vi "VisualCheck2.vi"(4 "Model":string="AVN", 6 "Slot":T1, 7 "ComPort":refnum<visa-resource-name>="COM1", 8 "error in":errorcluster, 10 "测试项":string="按键") -> (0 "error out":errorcluster, 3 "StringOut":string="ÿÿÿÿÿÿÿÿÿÿÿÿÿÿÿÿÿÿÿÿÿÿÿÿÿÿÿ")   [LabVIEW 2013]
uses:
  SystemCode/SysControl/Slot.ctl
  <vilib>/Utility/miscctls.llb/LVBoundsTypeDef.ctl
  C:/Program Files/National Instruments/LabVIEW 2013/examples/Instrument IO/Serial/support/Serial - Settings.ctl
  <vilib>/DAQmx/read.llb/DAQmx Read (Digital 1D Bool NChan 1Samp 1Line).vi
  GlobalValue.vi
  <vilib>/Instr/_visa.llb/VISA Configure Serial Port (Instr).vi
  <vilib>/DAQmx/create/channels.llb/DAQmx Create Channel (DI-Digital Input).vi
  <vilib>/DAQmx/miscellaneous.llb/DAQmx Fill In Error Info.vi
panel:
  in  "StopRef":refnum<vi>
  out "STOP2":bool
  out "按键2":T2 {"TUNE" scale=0.0..10.0}
  out "按键1":T3 {"VOL" scale=0.0..10.0}
  out "STOP":bool
  out "按键结果":bool
  out "TUNE按下":bool=TRUE
  out "TUNE旋转":bool=TRUE
  out "VOL旋转":bool=TRUE
  out "VOL按下":bool=TRUE
  out "FAIL":bool
  out "PASS":bool
  out "状态":string
  out "DVD仓":picture
  out "屏幕":picture
  in  "Debug":bool
  out "反馈结果":bool
  out "对比字符串":string
  in  "测试项目":u16(ring) items=["Reset", "按键", "倒车视频", "倒车视频", "按键灯亮", "DVD灯光红色", "DVD灯光蓝色", "按键灯亮", "入碟", "放入CD碟", "放入DVD碟", "出碟", "换碟", "视频播放", "拔除USB1", "拔除USB", "拔除导航卡", "拔除SD卡"]
  out "Result":bool
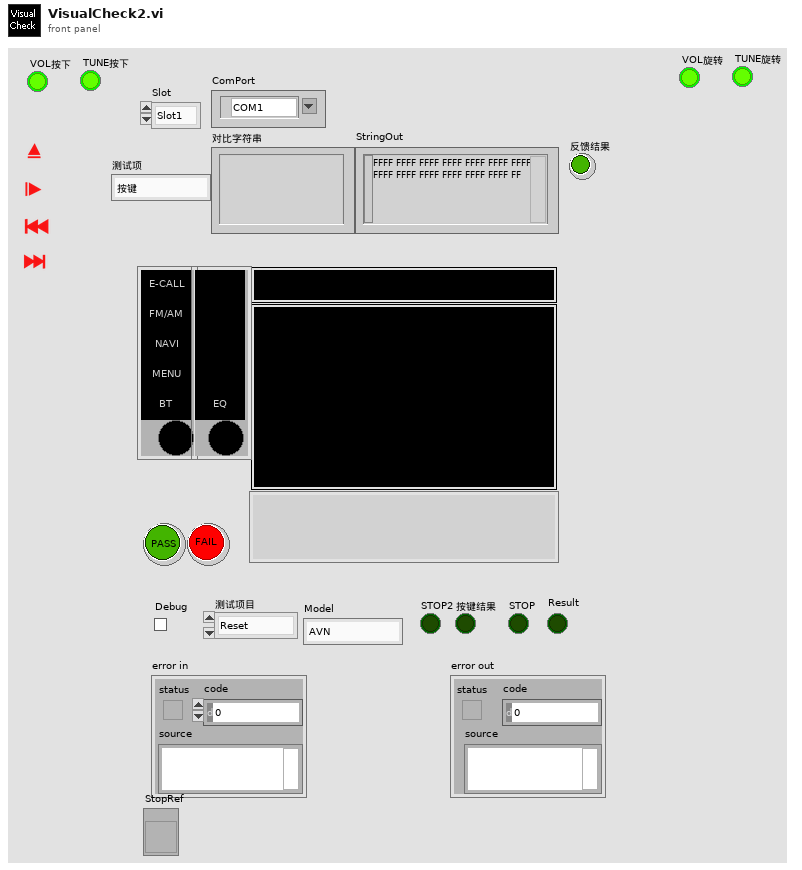
[diagram p1: front panel]
types:
  T1 = typedef "Slot.ctl" = enum16{"Slot1", "Slot2", "Slot3", "Slot4"}
  T2 = cluster{"EJECT":bool, "PLAY/PAUSE":bool, "PREV":bool, "NEXT":bool, "EQ":bool, "SRC":bool, "TUNE":dbl, "SEL":bool}
  T3 = cluster{"ECALL":bool, "FM/AM":bool, "NAVI":bool, "MENU":bool, "BT":bool, "DVD":bool, "VOL":dbl, "AUXIN":bool}
  T4 = typedef "Serial - Settings.ctl" = cluster{"波特率":u32, "数据比特":u16, "奇偶":enum16{"None", "Odd", "Even", "Mark", "Space"}, "停止位":u16, "流控制":u16}
  T5 = typedef "LVBoundsTypeDef.ctl" = cluster{"Width":u32, "Height":u32}
  T6 = typedef "DAQConfig.ctl" = cluster{"DIO":string[][], "AO":string[][], "AI":string[][]}
  T7 = typedef "imagedata.ctl" = cluster{"image type":i32, "image depth":i32, "image":u8[], "mask":u8[], "colors":u32[], "Rectangle":cluster{"left":i16, "top":i16, "right":i16, "bottom":i16}}
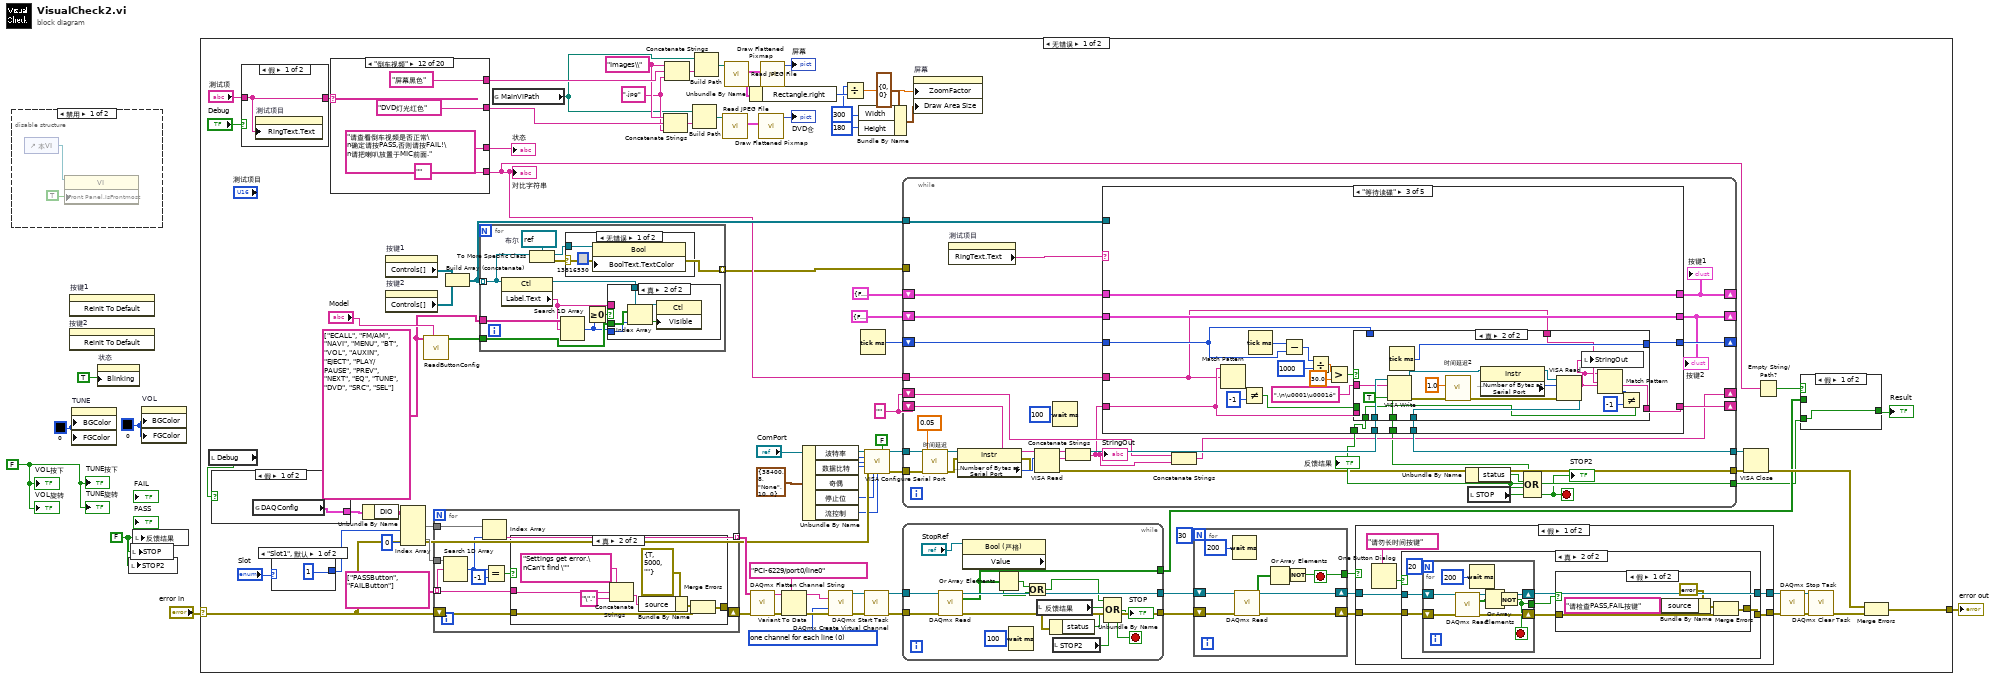
[diagram p0: block diagram]
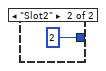
[diagram p3: hidden frame]
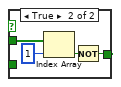
[diagram p4: hidden frame]
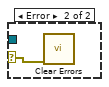
[diagram p5: hidden frame]
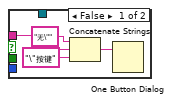
[diagram p6: hidden frame]
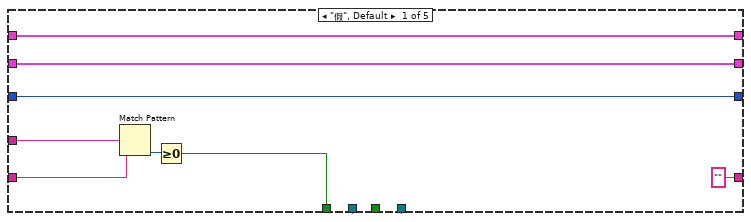
[diagram p7: hidden frame]
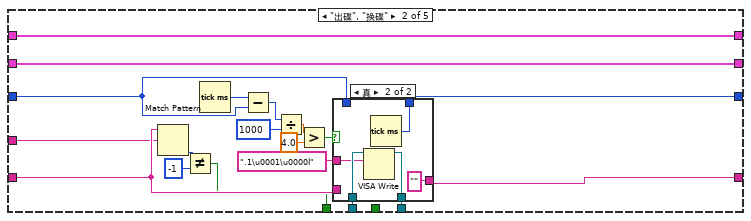
[diagram p8: hidden frame]
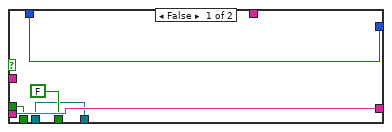
[diagram p10: hidden frame]
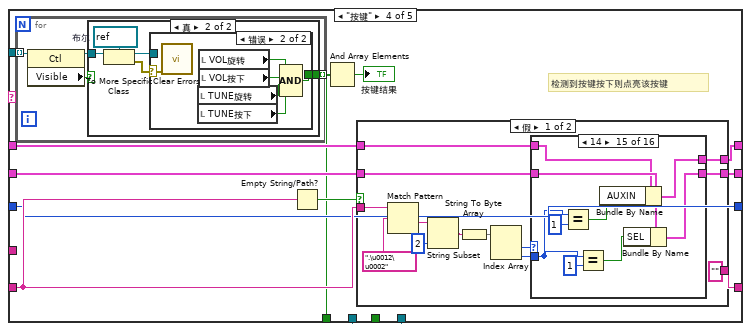
[diagram p11: hidden frame]
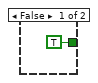
[diagram p12: hidden frame]
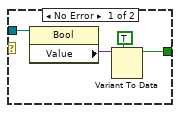
[diagram p13: hidden frame]
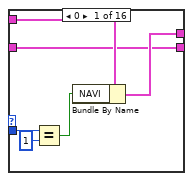
[diagram p14: hidden frame]
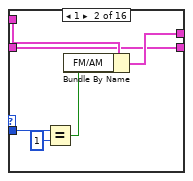
[diagram p15: hidden frame]
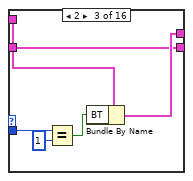
[diagram p16: hidden frame]
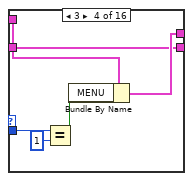
[diagram p17: hidden frame]
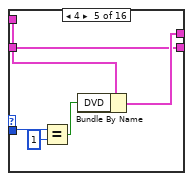
[diagram p18: hidden frame]
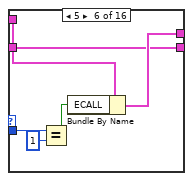
[diagram p19: hidden frame]
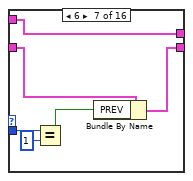
[diagram p20: hidden frame]
diagram:
  w4 = u32 0 ("颜色盒 3")
  w3 = u32 0 ("颜色盒 3")
  w1 = FALSE ("STOP")
  w2 = FALSE ("E-CALL")
  n1 = disable-structure shown="禁用" {
    frame Disabled {
      n2 = control-ref of="本VI"() -> (w9:refnum<vi>)
      n3 = property class="VI"(reference=w9, "Front Panel.IsFrontmost"=TRUE ("前面板窗口:在最前")) -> ()  [unwired: 1 in, 2 out]
    }
    frame Enabled {
    }
  }
  n4 = invoke on="按键1" class="Clust" method="Reinit To Default"() -> ()  [unwired: 3 in, 3 out]
  n5 = invoke on="按键2" class="Clust" method="Reinit To Default"() -> ()  [unwired: 3 in, 3 out]
  n6 = property on="TUNE" class="Knob (严格)"("BGColor"=w4, "FGColor"=w4) -> ()  [unwired: 2 in, 2 out]
  n7 = property on="状态" class="Str"("Blinking"=TRUE ("闪烁")) -> ()  [unwired: 2 in, 2 out]
  n8 = local write "STOP2"(w1) -> ()
  n9 = local write "STOP"(w1) -> ()
  n10 = local write "反馈结果"(w1) -> ()
  n11 = property on="VOL" class="Knob (严格)"("BGColor"=w3, "FGColor"=w3) -> ()  [unwired: 2 in, 2 out]
  n12 = case shown="无错误" "error in" {
    selector: "error in" -> [w56 w555]
    tunnel: [w23 w555] -> w6
    frame No Error {
      w28 = string[] ["ECALL", "FM/AM", "NAVI", "MENU", "BT", "VOL", "AUXIN", "EJECT", "PLAY/PAUSE", "PREV", "NEXT", "EQ", "TUNE", "DVD", "SRC", "SEL"] ("数组 2")
      w22 = ""
      w68 = u32 300 ("Width")
      w54 = ".jpg" ("字符串")
      w55 = "Images\\" ("名称或相对路径")
      w84 = 0 items=["one channel for each line", "one channel for all lines"] ("line grouping")
      n13 = local read "Debug"() -> (w44:bool)
      n14 = case shown="假" w44 {
        tunnel: [w397 w398] -> w83
        frame False {
          n15 = global read "GlobalValue.vi" "DAQConfig"() -> (w397:T6)
        }
        frame True {
          n16 = call "ReadDAQConfig.vi"() -> ("DAQConfig"=w398:T6)  [unwired: 10 in, 1 out]
        }
      }
      n17 = case shown="假" "Debug" {
        tunnel: [w438 w439] -> w75
        tunnel: "测试项" -> [w438 _]
        frame False {
          n18 = property on="测试项目" class="Ring (严格)"("RingText.Text"=w438) -> ()  [unwired: 2 in, 2 out]
        }
        frame True {
          n19 = property on="测试项目" class="Ring (严格)"() -> ("RingText.Text"=w439:string)  [unwired: 2 in, 2 out]
        }
      }
      n20 = case shown="\"Slot1\", 默认" "Slot" {
        tunnel: [1 ("索引 (行)") 2 ("索引 (行)")] -> w15
        frame "Slot1", Default {
        }
        frame "Slot2" {
        }
      }
      n21 = case shown="\"倒车视频\"" w75 {
        selector: w75 -> [_ _ _ _ _ _ _ _ _ _ _ _ _ _ _ _ w506 _ _ _]
        tunnel: ["屏幕黑色" ("ImageName") "屏幕黑色" ("ImageName") "屏幕黑色" ("ImageName") "屏幕黑色" ("ImageName") "屏幕黑色" ("ImageName") "屏幕黑色" ("ImageName") "屏幕黑色" ("ImageName") "屏幕黑色" ("ImageName") "屏幕黑色" ("ImageName") "屏幕黑色" ("ImageName") "屏幕黑色" ("ImageName") "屏幕黑色" ("ImageName") "屏幕黑色" ("ImageName") "屏幕黑色" ("ImageName") "屏幕黑色" ("ImageName") "屏幕黑色" ("ImageName") "屏幕黑色" ("ImageName") "屏幕校准" ("ImageName") "屏幕黑色" ("ImageName") "屏幕黑色" ("ImageName")] -> w65
        tunnel: ["DVD灯光红色" ("字符串") "DVD灯光蓝色" ("字符串") "DVD灯光蓝色" ("字符串") "DVD灯光蓝色" ("字符串") "DVD灯光蓝色" ("字符串") "DVD灯光红色" ("字符串") "DVD灯光红色" ("字符串") "DVD灯光红色" ("字符串") "DVD灯光红色" ("字符串") "DVD灯光红色" ("字符串") "入碟" ("字符串") "DVD灯光红色" ("字符串") "入碟" ("字符串") "DVD灯光红色" ("字符串") "入碟" ("字符串") "入碟" ("字符串") "DVD灯光蓝色" ("字符串") "DVD灯光蓝色" ("字符串") "入碟" ("字符串") "DVD灯光红色" ("字符串")] -> w74
        tunnel: ["DVD灯光为红色\n确定按PASS,否则按FAIL" ("字符串") "DVD灯光为蓝色\n确定按PASS,否则按FAIL" ("字符串") "请按下RST复位按键\n确定按PASS,否则按FAIL" ("字符串") "请查看地图版本是否正确\n确定按PASS,否则按FAIL" ("字符串") "请依次按下按键!\n如按键有问题请按FAIL." ("字符串") "请查看按键灯是否全亮!\n确定请按PASS,否则请按FAIL." ("字符串") "请拔掉SD卡!" ("字符串") "请拔掉导航卡!" ("字符串") "请拔掉USB!" ("字符串") "请拔掉USB1!" ("字符串") "请查看碟片状态是否正常出碟!\n确定请按PASS,否则请按FAIL" ("字符串") "请查看倒车视频是否正常\n确定请按PASS,否则请按FAIL!\n请把喇叭放置于MIC前面." ("字符串") "请放入CD测试碟!" ("字符串") "等待读碟!" ("字符串") "请放入DVD测试碟!" ("字符串") "请更换DVD碟!" ("字符串") w504 "请校准屏幕!" ("字符串") "请放入测试碟!" ("字符串") "请查看视频播放和分枕屏是否正常\n确定请按PASS,否则请按FAIL!" ("字符串")] -> w57
        tunnel: ["" ("字符串") "" ("字符串") "" ("字符串") "" ("字符串") "ÿ" ("字符串") "" ("字符串") ".\f\u0002\u0000\u0000" ("字符串") ".9\u0002\u0000\u0000" ("字符串") ".\u000e\u0002\u0000\u0000" ("字符串") ".\u0010\u0002\u0000\u0000" ("字符串") ".\n\u0002\u0000\u0000" ("字符串") "" ("字符串") ".\n\u0002\u0000\u0001" ("字符串") ".\n\u0002\u0001\u0002" ("字符串") ".\n\u0002\u0000\u0001" ("字符串") ".\n\u0002\u0000\u0000" ("字符串") "ÿÿ" ("字符串") ".\u0003\u0002\b\u0000ò" ("字符串") ".\n\u0002\u0000\u0001" ("字符串") "" ("字符串")] -> w21
        frame "DVD灯光红色" {
        }
        frame "DVD灯光蓝色" {
        }
        frame "Reset" {
        }
        frame "查看地图版本" {
        }
        frame "按键" {
        }
        frame "按键灯亮" {
          (unwired) TRUE ("可见")
        }
        frame "拔除SD卡" {
        }
        frame "拔除导航卡" {
        }
        frame "拔除USB" {
        }
        frame "拔除USB1" {
        }
        frame "出碟" {
        }
        frame "倒车视频" {
        }
        frame "放入CD碟" {
        }
        frame "等待读碟" {
        }
        frame "放入DVD碟" {
        }
        frame "换碟" {
        }
        frame "空", Default {
          n22 = Concatenate Strings("无“" ("字符串"), w506, "”测试项目" ("字符串")) -> (w504:string)
        }
        frame "屏幕校准" {
        }
        frame "入碟" {
        }
        frame "视频播放" {
        }
      }
      "状态" <- w57
      "对比字符串" <- w21
      n23 = Unbundle By Name(w83) -> ("DIO"=w81:string[][])
      n24 = property on="按键1" class="Clust"() -> ("Controls[]"=w29:refnum<vi>[])  [unwired: 2 in, 2 out]
      n25 = property on="按键2" class="Clust"() -> ("Controls[]"=w27:refnum<vi>[])  [unwired: 2 in, 2 out]
      n26 = Index Array(array=w81, index (col) #1=w15, index (col) #2=0 ("索引 (列)")) -> (element #1=w79:string[], element #2=w80:string[])  [unwired: 2 in]
      n27 = call "ReadButtonConfig.vi"("section"="Model", "数组 2"=w28) -> ("数组"=w10:bool[])  [unwired: 9 in]
      n28 = for {
        tunnel: string[] ["PASSButton", "FAILButton"] -> [w545] mode=indexing
        tunnel: w80 -> [w541]
        tunnel: w79 -> [w540]
        shift-right: [w538] -> w78
        shift-left: w56 -> [w539]
        tunnel: [w537] -> w76 mode=indexing
        n29 = Search 1D Array(1D array=w541, element=w545) -> (index of element=w542:i32)  [unwired: 1 in]
        n30 = Index Array(array=w540, index=w542) -> (element=w537:string)
        n31 = Equal?(x=w542, y=-1) -> (x = y?=w544:bool)
        n32 = case shown="真" w544 {
          tunnel: w545 -> [_ w550]
          tunnel: w539 -> [w546 w549]
          tunnel: [w546 w548] -> w538
          frame False {
          }
          frame True {
            n33 = Concatenate Strings("Settings get error.\nCan't find \"" ("message"), w550, "\"." ("string")) -> (w553:string)
            n34 = Bundle By Name(cluster=errorcluster {"status"=TRUE, "code"=5000, "source"=""} ("error in 1 (no error)"), "source"=w553) -> (w552:errorcluster)
            n35 = Merge Errors(w552, w549) -> (w548:errorcluster)
          }
        }
      }
      n36 = Build Array (concatenate)(w29, w27) -> (w26:refnum<vi>[])
      n37 = for {
        tunnel: w28 -> [w112]
        tunnel: w10 -> [w110]
        tunnel: w26 -> [w105] mode=indexing
        tunnel: [w103] -> w12 mode=indexing
        w109 = refnum<vi> refnum  # 布尔
        n38 = property class="Ctl"(reference=w105) -> (reference out=w106:refnum<vi>, "Label.Text"=w104:string)  [unwired: 1 in, 1 out]
        n39 = To More Specific Class(target class=w109, reference=w105) -> (specific class reference=w108:refnum<vi>, error out=w103:errorcluster)  [unwired: 1 in]
        n40 = Search 1D Array(1D array=w112, element=w104) -> (index of element=w107:i32)  [unwired: 1 in]
        n41 = case shown="无错误" w103 {
          selector: w103 -> [_ w115]
          tunnel: w108 -> [w113 _]
          frame No Error {
            n42 = property class="Bool"(reference=w113, "BoolText.TextColor"=u32 13816530 ("颜色盒")) -> ()  [unwired: 1 in, 2 out]
          }
          frame Error {
            n43 = call <vilib>:"Clear Errors.vi"("error in (no error)"=w115) -> ()  [unwired: 6 in, 1 out]
          }
        }
        n44 = Greater Or Equal To 0?(x=w107) -> (x >= 0?=w111:bool)
        n45 = case shown="真" w111 {
          tunnel: w110 -> [_ w122]
          tunnel: w106 -> [_ w123]
          tunnel: w107 -> [_ w121]
          tunnel: w104 -> [w118 _]
          frame False {
            n46 = Concatenate Strings("无\"" ("消息"), w118, "\"按键" ("字符串")) -> (w116:string)
            n47 = One Button Dialog(message=w116) -> ()  [unwired: 1 in, 1 out]
          }
          frame True {
            n48 = Index Array(array=w122, index=w121) -> (element=w120:bool)
            n49 = property class="Ctl"(reference=w123, "Visible"=w120) -> ()  [unwired: 1 in, 2 out]
          }
        }
      }
      n50 = global read "GlobalValue.vi" "MainViPath"() -> (w11:path)
      n51 = Concatenate Strings(w55, w74, w54) -> (w73:string)
      n52 = Concatenate Strings(w55, w65, w54) -> (w63:string)
      n53 = Build Path(base path=w11, name or relative path=w73) -> (appended path=w72:path)
      n54 = Build Path(base path=w11, name or relative path=w63) -> (appended path=w64:path)
      n55 = call <vilib>:"Read JPEG File.vi"("path to JPEG file"=w72) -> ("image data"=w71:T7)  [unwired: 8 in, 2 out]
      n56 = call <vilib>:"Read JPEG File.vi"("path to JPEG file"=w64) -> ("image data"=w66:T7)  [unwired: 8 in, 2 out]
      n57 = Unbundle By Name(w66) -> ("Rectangle.right"=w69:i16)
      n58 = call <vilib>:"DAQmx Flatten Channel String.vi"("names in"=w76, "error in"=w78) -> ("names out"=w88:string, "error out"=w86:errorcluster)  [unwired: 12 in]
      n59 = call <vilib>:"Draw Flattened Pixmap.vi"("image data"=w71) -> ("new picture"=→"DVD仓":picture)  [unwired: 8 in]
      n60 = call <vilib>:"Draw Flattened Pixmap.vi"("image data"=w66) -> ("new picture"=→"屏幕":picture)  [unwired: 8 in]
      n61 = Variant To Data(error in=w86, type=tag "PCI-6229/port0/line0" ("lines"), Variant=w88) -> (data=w87:tag, error out=w85:errorcluster)
      n62 = Unbundle By Name(T4 {"波特率"=38400, "数据比特"=8, "奇偶"=enum."None", "停止位"=10, "流控制"=0} ("串口设置")) -> ("波特率"=w38:u32, "数据比特"=w39:u16, "奇偶"=w40:enum16{"None", "Odd", "Even", "Mark", "Space"}, "停止位"=w41:u16, "流控制"=w36:u16)
      n63 = call-poly <vilib>:"DAQmx Create Virtual Channel.vi"("lines"=w87, "line grouping"=w84, "error in"=w85) -> ("task out"=w95:refnum<k21>, "error out"=w94:errorcluster)  [unwired: 11 in]
      n64 = Divide(x=w68, y=w69) -> (x/y=w60:dbl)
      n65 = Bundle By Name(cluster=T5 {"Width"=0, "Height"=0} ("绘图区域大小"), "Width"=w68, "Height"=u32 180) -> (w59:T5)
      n66 = Tick Count (ms)() -> (millisecond timer value=w32:u32)
      n67 = call <vilib>:"DAQmx Start Task.vi"("task/channels in"=w95, "error in"=w94) -> ("task out"=w93:refnum<k21>, "error out"=w92:errorcluster)  [unwired: 12 in]
      n68 = call-poly "VISA Configure Serial Port"("VISA resource name"="ComPort", "Enable Termination\nChar (T)"=FALSE ("Enable Termination\nChar (T)"), "baud rate (9600)"=w38, "data bits (8)"=w39, "parity (0:none)"=w40, "error in (no error)"=w56, "stop bits (10: 1 bit)"=w41, "flow control (0:none)"=w36) -> ("VISA resource name out"=w34:refnum<visa-resource-name>, "error out"=w33:errorcluster)  [unwired: 2 in, 4 out]
      n69 = while {
        tunnel: w34 -> [w143]
        tunnel: w33 -> [w140]
        tunnel: [w149] -> w31
        tunnel: [w128] -> w43
        shift-right: [w151] -> _
        shift-left: w22 -> [w154]
        tunnel: w21 -> [w146]
        shift-right: [w148] -> _
        shift-left: w32 -> [w147]
        tunnel: [w145] -> w18
        tunnel: w26 -> [w138]
        shift-right: [w134] -> _
        shift-left: T3 {"ECALL"=FALSE, "FM/AM"=FALSE, "NAVI"=FALSE, "MENU"=FALSE, "BT"=FALSE, "DVD"=FALSE, "VOL"=0.0, "AUXIN"=FALSE} ("按键1 2") -> [w137]
        shift-right: [w135] -> _
        shift-left: T2 {"EJECT"=FALSE, "PLAY/PAUSE"=FALSE, "PREV"=FALSE, "NEXT"=FALSE, "EQ"=FALSE, "SRC"=FALSE, "TUNE"=0.0, "SEL"=FALSE} ("按键2") -> [w136]
        shift-right: [w129] -> _
        shift-left: w22 -> [w131]
        tunnel: w12 -> [_]
        stop <- w126 stop-if-true
        n70 = call "时间延迟"("error in (no error)"=w140, "Delay Time (s)"=0.05) -> ("error out"=w139:errorcluster)  [unwired: 9 in]
        n71 = property on="测试项目" class="Ring (严格)"() -> ("RingText.Text"=w152:string)  [unwired: 2 in, 2 out]
        n72 = property class="Instr"(reference=w143, error in=w139) -> (reference out=w142:refnum<visa-resource-name>, error out=w141:errorcluster, "Serial Settings:Number of Bytes at Serial Port"=w144:u32)
        n73 = VISA Read(VISA resource name=w142, byte count=w144, error in (no error)=w141) -> (VISA resource name out=w150:refnum<visa-resource-name>, read buffer=w153:string, error out=w128:errorcluster)  [unwired: 1 out]
        n74 = Wait (ms)(milliseconds to wait=u32 100 ("等待时间（毫秒）")) -> ()  [unwired: 1 out]
        n75 = Concatenate Strings(w154, w153) -> (w130:string)
        "StringOut" <- w130
        n76 = case shown="\"等待读碟\"" w152 {
          tunnel: w130 -> [w159 w168 w201 w243 w389]
          tunnel: ["" w179 w194 w244 w389] -> w151
          tunnel: w150 -> [w163 w182 w196 w241 w388]
          tunnel: [w163 w181 w197 w241 w388] -> w149
          tunnel: [w162 w175 w208 w240 w387] -> w148
          tunnel: w147 -> [w162 w174 w207 w240 w387]
          tunnel: [w156 w166 w191 w234 _] -> w145
          tunnel: w146 -> [w158 w167 w193 _ _]
          tunnel: w138 -> [_ _ _ w233 w384]
          tunnel: [w161 w165 w200 w239 w386] -> w134
          tunnel: [w160 w164 w199 w238 w385] -> w135
          tunnel: w137 -> [w161 w165 w200 w237 w386]
          tunnel: w136 -> [w160 w164 w199 w236 w385]
          tunnel: [_ _ w198 _ _] -> w125
          frame "假", Default {
            n77 = Match Pattern(string=w159, regular expression=w158) -> (offset past match=w157:i32)  [unwired: 1 in, 3 out]
            n78 = Greater Or Equal To 0?(x=w157) -> (x >= 0?=w156:bool)
          }
          frame "出碟", "换碟" {
            n79 = Match Pattern(string=w168, regular expression=w167) -> (offset past match=w170:i32)  [unwired: 1 in, 3 out]
            n80 = Not Equal?(x=w170, y=-1) -> (x != y?=w166:bool)
            n81 = Tick Count (ms)() -> (millisecond timer value=w178:u32)
            n82 = Subtract(x=w178, y=w174) -> (x-y=w177:u32)
            n83 = Divide(x=w177, y=u32 1000) -> (x/y=w173:dbl)
            n84 = Greater?(x=w173, y=4.0) -> (0:w171:bool)
            n85 = case shown="真" w171 {
              tunnel: w182 -> [w185 w190]
              tunnel: [w185 w189] -> w181
              tunnel: ".1\u0001\u0000Í" ("写入缓冲区") -> [_ w188]
              tunnel: [w183 ""] -> w179
              tunnel: [w184 w186] -> w175
              tunnel: w174 -> [w184 _]
              tunnel: w168 -> [w183 _]
              frame False {
              }
              frame True {
                n86 = VISA Write(VISA resource name=w190, write buffer=w188) -> (VISA resource name out=w189:refnum<visa-resource-name>)  [unwired: 1 in, 2 out]
                n87 = Tick Count (ms)() -> (millisecond timer value=w186:u32)
              }
            }
          }
          frame "等待读碟" {
            n88 = Match Pattern(string=w201, regular expression=w193) -> (offset past match=w203:i32)  [unwired: 1 in, 3 out]
            n89 = Not Equal?(x=w203, y=-1) -> (x != y?=w192:bool)
            n90 = Tick Count (ms)() -> (millisecond timer value=w211:u32)
            n91 = Subtract(x=w211, y=w207) -> (x-y=w210:u32)
            n92 = Divide(x=w210, y=u32 1000) -> (x/y=w206:dbl)
            n93 = Greater?(x=w206, y=30.0) -> (0:w204:bool)
            n94 = case shown="真" w204 {
              tunnel: [w215 w217] -> w194
              tunnel: [w216 w232] -> w208
              tunnel: w207 -> [w216 _]
              tunnel: w201 -> [w215 _]
              tunnel: [FALSE ("值(信号)") TRUE ("值(信号)")] -> w198
              tunnel: [w213 w225] -> w197
              tunnel: w196 -> [w213 w230]
              tunnel: ".\n\u0001\u0001ó" ("命令") -> [_ w229]
              tunnel: w193 -> [_ w222]
              tunnel: w192 -> [w212 _]
              tunnel: [w212 w221] -> w191
              frame False {
              }
              frame True {
                n95 = VISA Write(VISA resource name=w230, write buffer=w229) -> (VISA resource name out=w219:refnum<visa-resource-name>, error out=w228:errorcluster)  [unwired: 1 in, 1 out]
                n96 = Tick Count (ms)() -> (millisecond timer value=w232:u32)
                n97 = call "时间延迟2"("error in (no error)"=w228, "Delay Time (s)"=1.0) -> ("error out"=w227:errorcluster)  [unwired: 9 in]
                n98 = property class="Instr"(reference=w219) -> (reference out=w220:refnum<visa-resource-name>, "Serial Settings:Number of Bytes at Serial Port"=w218:u32)  [unwired: 1 in, 1 out]
                n99 = VISA Read(VISA resource name=w220, byte count=w218, error in (no error)=w227) -> (VISA resource name out=w225:refnum<visa-resource-name>, read buffer=w217:string)  [unwired: 2 out]
                n100 = local write "StringOut"(w217) -> ()
                n101 = Match Pattern(string=w217, regular expression=w222) -> (offset past match=w223:i32)  [unwired: 1 in, 3 out]
                n102 = Not Equal?(x=w223, y=-1) -> (x != y?=w221:bool)
              }
            }
          }
          frame "按键" {
            # "检测到按键按下则点亮该按键"
            n103 = for {
              tunnel: w233 -> [w248] mode=indexing
              tunnel: [w245] -> w235 mode=indexing
              n104 = property class="Ctl"(reference=w248) -> (reference out=w246:refnum<vi>, "Visible"=w247:bool)  [unwired: 1 in, 1 out]
              n105 = case shown="真" w247 {
                tunnel: w246 -> [_ w253]
                tunnel: [TRUE ("VOL按下") w251] -> w245
                frame False {
                }
                frame True {
                  w254 = refnum<vi> refnum  # 布尔
                  n106 = To More Specific Class(target class=w254, reference=w253) -> (specific class reference=w252:refnum<vi>, error out=w250:errorcluster)  [unwired: 1 in]
                  n107 = case shown="错误" w250 {
                    selector: w250 -> [_ w264]
                    tunnel: w252 -> [w258 _]
                    tunnel: [w255 w259] -> w251
                    frame No Error {
                      n108 = property class="Bool"(reference=w258) -> ("Value"=w257:variant)  [unwired: 1 in, 2 out]
                      n109 = Variant To Data(type=TRUE ("VOL按下"), Variant=w257) -> (data=w255:bool)  [unwired: 1 in, 1 out]
                    }
                    frame Error {
                      n110 = call <vilib>:"Clear Errors.vi"("error in (no error)"=w264) -> ()  [unwired: 6 in, 1 out]
                      n111 = local read "TUNE旋转"() -> (w261:bool)
                      n112 = local read "TUNE按下"() -> (w260:bool)
                      n113 = local read "VOL旋转"() -> (w263:bool)
                      n114 = local read "VOL按下"() -> (w262:bool)
                      n115 = Compound Arithmetic op=AND(w263, w262, w261, w260) -> (w259:bool)
                    }
                  }
                }
              }
            }
            n116 = Empty String/Path?(string/path=w243) -> (empty?=w242:bool)
            n117 = And Array Elements(Boolean array=w235) -> (logical AND=w234:bool)
            "按键结果" <- w234
            n118 = case shown="假" w242 {
              tunnel: ["" w383] -> w244
              tunnel: w243 -> [w270 w383]
              tunnel: w237 -> [w268 w381]
              tunnel: [w267 w381] -> w239
              tunnel: [w266 w382] -> w238
              tunnel: w236 -> [w265 w382]
              frame False {
                n119 = Match Pattern(string=w270, regular expression=".\u0012\u0002") -> (after substring=w271:string)  [unwired: 1 in, 3 out]
                n120 = String Subset(string=w271, length (rest)=2 ("长度（剩余）")) -> (substring=w275:string)  [unwired: 1 in]
                n121 = String To Byte Array(string=w275) -> (unsigned byte array=w274:u8[])
                n122 = Index Array(array=w274) -> (element #1=w273:u8, element #2=w272:u8)  [unwired: 2 in]
                n123 = case shown="14" w273 {
                  tunnel: w272 -> [w282 w288 w294 w300 w306 w312 w318 w324 w329 w339 w350 w356 w362 w368 w370 _]
                  tunnel: w268 -> [w280 w287 w292 w299 w305 w310 w315 w321 w326 w336 w347 w353 w359 w365 w372 w379]
                  tunnel: [w279 w286 w291 w298 w304 w309 w315 w321 w326 w336 w347 w353 w359 w365 w371 w379] -> w267
                  tunnel: [w278 w284 w290 w296 w302 w308 w316 w322 w328 w338 w349 w355 w361 w367 w377 w380] -> w266
                  tunnel: w265 -> [w278 w284 w290 w296 w302 w308 w314 w320 w328 w338 w346 w352 w358 w364 w375 w380]
                  frame 0 {
                    n124 = Equal?(x=w282, y=u8 1) -> (x = y?=w281:bool)
                    n125 = Bundle By Name(cluster=w280, "NAVI"=w281) -> (w279:T3)
                  }
                  frame 1 {
                    n126 = Equal?(x=w288, y=u8 1) -> (x = y?=w285:bool)
                    n127 = Bundle By Name(cluster=w287, "FM/AM"=w285) -> (w286:T3)
                  }
                  frame 2 {
                    n128 = Equal?(x=w294, y=u8 1) -> (x = y?=w293:bool)
                    n129 = Bundle By Name(cluster=w292, "BT"=w293) -> (w291:T3)
                  }
                  frame 3 {
                    n130 = Equal?(x=w300, y=u8 1) -> (x = y?=w297:bool)
                    n131 = Bundle By Name(cluster=w299, "MENU"=w297) -> (w298:T3)
                  }
                  frame 4 {
                    n132 = Equal?(x=w306, y=u8 1) -> (x = y?=w303:bool)
                    n133 = Bundle By Name(cluster=w305, "DVD"=w303) -> (w304:T3)
                  }
                  frame 5 {
                    n134 = Equal?(x=w312, y=u8 1) -> (x = y?=w311:bool)
                    n135 = Bundle By Name(cluster=w310, "ECALL"=w311) -> (w309:T3)
                  }
                  frame 6 {
                    n136 = Equal?(x=w318, y=u8 1) -> (x = y?=w317:bool)
                    n137 = Bundle By Name(cluster=w314, "PREV"=w317) -> (w316:T2)
                  }
                  frame 7 {
                    n138 = Equal?(x=w324, y=u8 1) -> (x = y?=w323:bool)
                    n139 = Bundle By Name(cluster=w320, "NEXT"=w323) -> (w322:T2)
                  }
                  frame 8 {
                    n140 = control-ref of="VOL"() -> (w327:refnum<vi>)
                    n141 = case shown="1" w329 {
                      tunnel: w327 -> [_ w332 w335]
                      frame 0, Default {
                      }
                      frame 1 {
                        n142 = property class="Knob (严格)"(reference=w332, "BGColor"=u32 6618880 ("颜色盒 3")) -> ()  [unwired: 1 in, 2 out]
                        n143 = local write "VOL按下"(TRUE ("VOL按下")) -> ()
                      }
                      frame 2, 3 {
                        n144 = property class="Knob (严格)"(reference=w335, "FGColor"=u32 6618880 ("颜色盒 3")) -> ()  [unwired: 1 in, 2 out]
                        n145 = local write "VOL旋转"(TRUE ("VOL按下")) -> ()
                      }
                    }
                  }
                  frame 9 {
                    n146 = control-ref of="TUNE"() -> (w337:refnum<vi>)
                    n147 = case shown="2, 3" w339 {
                      tunnel: w337 -> [_ w342 w345]
                      frame 0, Default {
                      }
                      frame 1 {
                        n148 = property class="Knob (严格)"(reference=w342, "BGColor"=u32 6618880 ("颜色盒 3")) -> ()  [unwired: 1 in, 2 out]
                        n149 = local write "TUNE按下"(TRUE ("VOL按下")) -> ()
                      }
                      frame 2, 3 {
                        n150 = property class="Knob (严格)"(reference=w345, "FGColor"=u32 6618880 ("颜色盒 3")) -> ()  [unwired: 1 in, 2 out]
                        n151 = local write "TUNE旋转"(TRUE ("VOL按下")) -> ()
                      }
                    }
                  }
                  frame 10 {
                    n152 = Equal?(x=w350, y=u8 1) -> (x = y?=w348:bool)
                    n153 = Bundle By Name(cluster=w346, "EQ"=w348) -> (w349:T2)
                  }
                  frame 11 {
                    # "0B"
                    n154 = Equal?(x=w356, y=u8 1) -> (x = y?=w354:bool)
                    n155 = Bundle By Name(cluster=w352, "PLAY/PAUSE"=w354) -> (w355:T2)
                  }
                  frame 12 {
                    n156 = Equal?(x=w362, y=u8 1) -> (x = y?=w360:bool)
                    n157 = Bundle By Name(cluster=w358, "EJECT"=w360) -> (w361:T2)
                  }
                  frame 13 {
                    n158 = Equal?(x=w368, y=u8 1) -> (x = y?=w366:bool)
                    n159 = Bundle By Name(cluster=w364, "SRC"=w366) -> (w367:T2)
                  }
                  frame 14 {
                    n160 = Equal?(x=w370, y=u8 1) -> (x = y?=w374:bool)
                    n161 = Equal?(x=w370, y=u8 1) -> (x = y?=w376:bool)
                    n162 = Bundle By Name(cluster=w372, "AUXIN"=w374) -> (w371:T3)
                    n163 = Bundle By Name(cluster=w375, "SEL"=w376) -> (w377:T2)
                  }
                  frame 20, Default {
                  }
                }
              }
              frame True {
              }
            }
          }
          frame "按键灯亮" {
            n164 = for {
              tunnel: w384 -> [w392] mode=indexing
              w390 = refnum<vi> refnum  # 布尔
              n165 = To More Specific Class(target class=w390, reference=w392) -> (specific class reference=w391:refnum<vi>, error out=w393:errorcluster)  [unwired: 1 in]
              n166 = case shown="无错误" w393 {
                selector: w393 -> [_ w396]
                tunnel: w391 -> [w394 _]
                frame No Error {
                  n167 = property class="Bool"(reference=w394, "BoolText.TextColor"=u32 16711680 ("颜色盒")) -> ()  [unwired: 1 in, 2 out]
                }
                frame Error {
                  n168 = call <vilib>:"Clear Errors.vi"("error in (no error)"=w396) -> ()  [unwired: 6 in, 1 out]
                }
              }
            }
          }
        }
        "反馈结果" <- w145
        "按键1" <- w134
        "按键2" <- w135
        n169 = Concatenate Strings(w131, w130) -> (w129:string)
        n170 = Unbundle By Name(w128) -> ("status"=w127:bool)
        n171 = local read "STOP"() -> (w133:bool)
        n172 = Compound Arithmetic op=OR(w125, w127, w145, w133) -> (w126:bool)
        "STOP2" <- w126
      }
      n173 = while {
        tunnel: [w532] -> w19
        tunnel: w93 -> [w536]
        tunnel: w92 -> [w535]
        tunnel: [w534] -> w52
        tunnel: [w530] -> w51
        stop <- w528 stop-if-true
        n174 = call-poly <vilib>:"DAQmx Read.vi"("task/channels in"=w536, "error in"=w535) -> ("task out"=w534:refnum<k21>, "data"=w532:bool[], "error out"=w530:errorcluster)  [unwired: 11 in]
        n175 = property class="Bool (严格)"(reference="StopRef") -> ("Value"=w523:bool)  [unwired: 1 in, 2 out]
        n176 = Or Array Elements(Boolean array=w532) -> (logical OR=w526:bool)
        n177 = Wait (ms)(milliseconds to wait=u32 100 ("等待时间（毫秒）")) -> ()  [unwired: 1 out]
        n178 = Or(x=w526, y=w523) -> (x .or. y?=w525:bool)
        n179 = local read "反馈结果"() -> (w531:bool)
        n180 = Unbundle By Name(w530) -> ("status"=w529:bool)
        n181 = local read "STOP2"() -> (w527:bool)
        n182 = Compound Arithmetic op=OR(w525, w531, w529, w527) -> (w528:bool)
        "STOP" <- w528
      }
      n183 = property on="屏幕" class="Pict"("ZoomFactor"=w60, "Draw Area Size"=w59) -> ()  [unwired: 2 in, 2 out]
      n184 = for {
        N: 30 -> [_]
        shift-right: [w436] -> w48
        shift-left: w52 -> [w437]
        shift-right: [w434] -> w47
        shift-left: w51 -> [w435]
        tunnel: [w430] -> w49
        stop <- w430 stop-if-true
        n185 = Wait (ms)(milliseconds to wait=u32 200 ("等待时间（毫秒）")) -> ()  [unwired: 1 out]
        n186 = call-poly <vilib>:"DAQmx Read.vi"("task/channels in"=w437, "error in"=w435) -> ("task out"=w436:refnum<k21>, "data"=w432:bool[], "error out"=w434:errorcluster)  [unwired: 11 in]
        n187 = Or Array Elements(Boolean array=w432) -> (logical OR=w433:bool)
        n188 = Not(x=w433) -> (.not. x?=w430:bool)
      }
      n189 = case shown="假" w49 {
        tunnel: w48 -> [w403 w429]
        tunnel: [w401 w429] -> w46
        tunnel: w47 -> [w402 w428]
        tunnel: [w399 w428] -> w45
        frame False {
          n190 = One Button Dialog(message="请勿长时间按键" ("消息")) -> (true=w400:bool)  [unwired: 1 in]
          n191 = case shown="真" w400 {
            tunnel: w403 -> [w406 w413]
            tunnel: w402 -> [w405 w412]
            tunnel: [w405 w407] -> w399
            tunnel: [w406 w411] -> w401
            frame False {
            }
            frame True {
              n192 = for {
                N: 20 -> [_]
                shift-right: [w426] -> w411
                shift-left: w413 -> [w427]
                shift-right: [w424] -> w408
                shift-left: w412 -> [w425]
                tunnel: [w420] -> w409
                stop <- w420 stop-if-true
                n193 = call-poly <vilib>:"DAQmx Read.vi"("task/channels in"=w427, "error in"=w425) -> ("task out"=w426:refnum<k21>, "data"=w422:bool[], "error out"=w424:errorcluster)  [unwired: 11 in]
                n194 = Wait (ms)(milliseconds to wait=u32 200 ("等待时间（毫秒）")) -> ()  [unwired: 1 out]
                n195 = Or Array Elements(Boolean array=w422) -> (logical OR=w423:bool)
                n196 = Not(x=w423) -> (.not. x?=w420:bool)
              }
              n197 = case shown="假" w409 {
                tunnel: w408 -> [w416 w419]
                tunnel: [w415 w419] -> w407
                frame False {
                  n198 = Bundle By Name(cluster=errorcluster {"status"=TRUE, "code"=5000, "source"=""} ("error in 1 (no error)"), "source"="请检查PASS,FAIL按键" ("message")) -> (w418:errorcluster)
                  n199 = Merge Errors(w418, w416) -> (w415:errorcluster)
                }
                frame True {
                }
              }
            }
          }
        }
        frame True {
        }
      }
      n200 = VISA Close(VISA resource name=w31, error in (no error)=w43) -> (error out=w25:errorcluster)
      n201 = Empty String/Path?(string/path=w21) -> (empty?=w20:bool)
      n202 = call <vilib>:"DAQmx Stop Task.vi"("task/channels in"=w46, "error in"=w45) -> ("task out"=w91:refnum<k21>, "error out"=w90:errorcluster)  [unwired: 12 in]
      n203 = case shown="假" w20 {
        tunnel: [w98 w100] -> w17
        tunnel: w19 -> [_ w99]
        tunnel: w18 -> [w98 _]
        frame False {
        }
        frame True {
          n204 = Index Array(array=w99, index=1 ("索引")) -> (element=w101:bool)
          n205 = Not(x=w101) -> (.not. x?=w100:bool)
        }
      }
      "Result" <- w17
      n206 = call <vilib>:"DAQmx Clear Task.vi"("task in"=w91, "error in"=w90) -> ("error out"=w24:errorcluster)  [unwired: 13 in]
      n207 = Merge Errors(w25, w24) -> (w23:errorcluster)
    }
    frame Error {
    }
  }
  "error out" <- w6
  "VOL按下" <- w2
  "VOL旋转" <- w2
  "TUNE按下" <- w2
  "TUNE旋转" <- w2
